vi "Read Name.vi"(8 "error in (no error)":errorcluster, 11 "IViewable In":refnum<class "IViewable.lvclass">) -> (0 "error out":errorcluster, 2 "Name":string, 3 "IViewable Out":refnum<class "IViewable.lvclass">)   [LabVIEW 2015, in "IViewable.lvlib" / "IViewable.lvclass"]
doc: "<License>\nCopyright © 2017 Composed Systems, LLC | All rights reserved\nwww.composed.io\n\nAuthor: Ethan Stern <ethan.stern@composed.io>\n\nThis software is provided \"AS IS\" WITHOUT WARRANTIES, either express or implied, AND IS FOR EDUCATIONAL PURPOSES ONLY.\n</License>"
uses:
  IViewable.lvclass
  IViewable.lvclass/IViewable.ctl
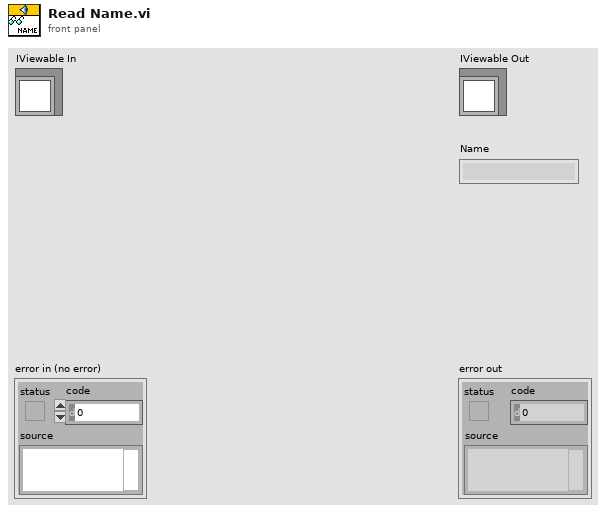
[diagram p1: front panel]
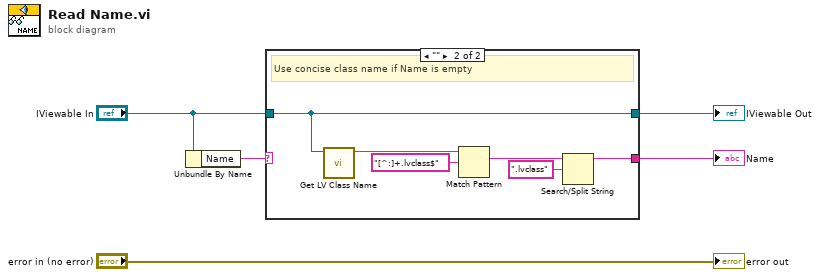
[diagram p0: block diagram]
diagram:
  n1 = Unbundle By Name("IViewable In") -> ("Name"=w1:string)
  n2 = case shown="\"\"" w1 {
    selector: w1 -> [w6 _]
    tunnel: [w6 w10] -> w2
    tunnel: "IViewable In" -> [w7 w8]
    tunnel: [w7 w8] -> w3
    frame "False", Default {
      # "Return assigned name"
    }
    frame "" {
      # "Use concise class name if Name is empty"
      n3 = call <vilib>:"Get LV Class Name.vi"("object"=w8) -> ("class name"=w9:string)  [unwired: 9 in, 1 out]
      n4 = Match Pattern(string=w9, regular expression="[^:]+.lvclass$") -> (match substring=w12:string)  [unwired: 1 in, 3 out]
      n5 = Search/Split String(string=w12, search string/char (-)=".lvclass") -> (substring before match=w10:string)  [unwired: 1 in, 2 out]
    }
  }
  "IViewable Out" <- w3
  "Name" <- w2
  "error out" <- "error in (no error)"
